vi "hama_orca_stop.vi"(8 "error in (no error)":errorcluster {"code" format="%.0x"}, 10 "Camera ON status":bool, 11 "Camera handle in":u32) -> (0 "error out":errorcluster {"code" format="%.0x"}, 2 "Camera ON":bool=TRUE, 3 "Camera handle out":u32)   [LabVIEW 2018]
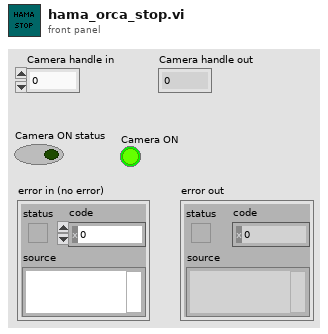
[diagram p1: front panel]
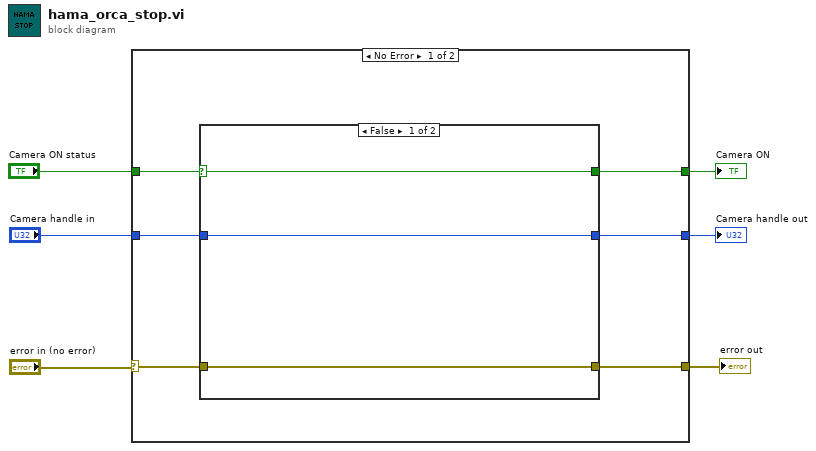
[diagram p0: block diagram]
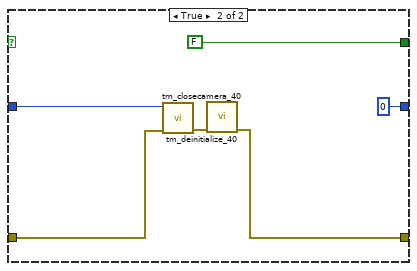
[diagram p2: hidden frame]
diagram:
  n1 = case shown="No Error" "error in (no error)" {
    selector: "error in (no error)" -> [w10 w24]
    tunnel: [w12 w24] -> w6
    tunnel: "Camera ON status" -> [w11 w23]
    tunnel: [w9 w22] -> w3
    tunnel: [w8 w23] -> w2
    tunnel: "Camera handle in" -> [w7 w22]
    frame No Error {
      n2 = case shown="False" w11 {
        selector: w11 -> [w15 _]
        tunnel: [w13 w17] -> w12
        tunnel: w10 -> [w13 w16]
        tunnel: [w14 u32 0 ("Camera Index")] -> w9
        tunnel: [w15 FALSE] -> w8
        tunnel: w7 -> [w14 w20]
        frame False {
        }
        frame True {
          n3 = call <userlib>:"tm_closecamera_40.vi"("error in (no error)"=w16, "Handle in"=w20) -> ("error out"=w19:errorcluster)  [unwired: 9 in]
          n4 = call <userlib>:"tm_deinitialize_40.vi"("error in (no error)"=w19) -> ("error out"=w17:errorcluster)  [unwired: 10 in]
        }
      }
    }
    frame Error {
    }
  }
  "error out" <- w6
  "Camera handle out" <- w3
  "Camera ON" <- w2
